vi "设置曲线属性.vi"(4 "监测曲线":refnum<vi>, 6 "XY图输入":refnum<vi>, 11 "曲线属性":cluster{"曲线名":string, "曲线颜色":u32, "线条宽度":u8}[](array[cluster])) -> ()   [LabVIEW 2020, in "数据显示.xctl"]
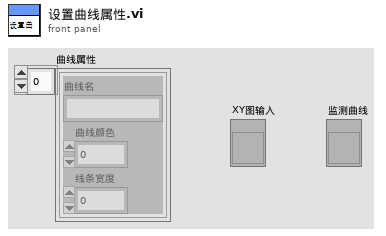
[diagram p1: front panel]
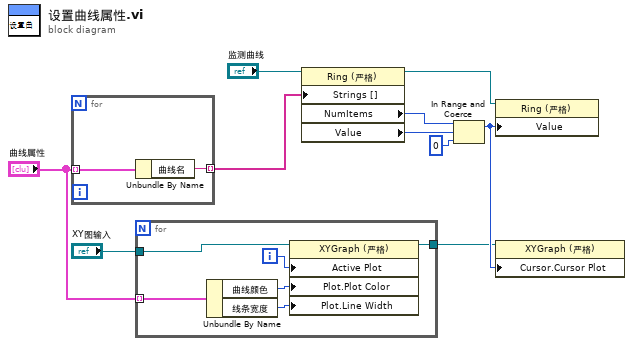
[diagram p0: block diagram]
diagram:
  n1 = for {
    tunnel: "曲线属性" -> [w12] mode=indexing
    tunnel: [w11] -> w1 mode=indexing
    n2 = Unbundle By Name(w12) -> ("曲线名"=w11:string)
  }
  n3 = for {
    tunnel: "曲线属性" -> [w17] mode=indexing
    tunnel: [w14] -> w5
    tunnel: "XY图输入" -> [w13]
    i -> [w18]
    n4 = Unbundle By Name(w17) -> ("曲线颜色"=w16:u32, "线条宽度"=w15:u8)
    n5 = property on="属性节点" class="XYGraph (严格)"(reference=w13, "Active Plot"=w18, "Plot.Plot Color"=w16, "Plot.Line Width"=w15) -> (reference out=w14:refnum<vi>)  [unwired: 1 in, 1 out]
  }
  n6 = property on="属性节点" class="Ring (严格)"(reference="监测曲线", "Strings []"=w1) -> (reference out=w7:refnum<vi>, "NumItems"=w4:u32, "Value"=w8:i32)  [unwired: 1 in, 1 out]
  n7 = In Range and Coerce(upper limit=w4, x=w8, lower limit=u32 0 ("下限")) -> (coerced(x)=w6:u32)  [unwired: 1 out]
  n8 = property on="属性节点" class="Ring (严格)"(reference=w7, "Value"=w6) -> ()  [unwired: 1 in, 2 out]
  n9 = property on="属性节点" class="XYGraph (严格)"(reference=w5, "Cursor.Cursor Plot"=w6) -> ()  [unwired: 1 in, 2 out]
